vi "RobotDriveOpen6MotorWithTalonSRX.vi"(0 "Left Motor 1":u8=255, 1 "Left Motor 2":u8=255, 2 "Left Motor 3":u8=255, 3 "Right Motor 1":u8=255, 4 "Right Motor 2":u8=255, 5 "Right Motor 3":u8=255, 7 "error in (no error)":errorcluster, 8 "Left Motor 1 Inverted":bool, 9 "Right Motor 1 Inverted":bool, 10 "Left Motor 2 Inverted":bool, 11 "Right Motor 2 Inverted":bool, 12 "Left Motor 3 Inverted":bool, 13 "Right Motor 3 Inverted":bool) -> (20 "RobotDriveDevRef":T1={"DevStatus"={"status"=FALSE, "code"=0, "source"=""}, "Motors[]"=[], "Square Inputs"=FALSE, "Max Output"=1.0}, 27 "error out":errorcluster)   [LabVIEW 2017, in "ArgosLib.lvlib"]
doc: "Opens a reference to the robot drive for a two-, four-, or six-motor robot using Talon SR motor controllers connected via CAN bus.\n\nFor 2-motor drive, connect Left Motor 1 and Right Motor 1.\nFor 4-motor drive, connect Left Motor 2 and Right Motor 2 in addition to the 2-motor drive connections.\nFor 6-motor drive, connect Left Motor 3 and Right Motor 3 in addition to the 4-motor drive connections.\n\nInversions are optional and are set to false if disconnected.\n\nThis software is licensed. Open the labview\\readme\\WPI Robotics Library Open Source License.txt file for more information."
uses:
  ArgosLib.lvlib
  <vilib>/Rock Robotics/WPI/RobotDrive/WPI_RobotDriveDevRef.ctl
  <vilib>/Rock Robotics/WPI/MotorControl/WPI_MotorControlDeviceRef.ctl
  <vilib>/Rock Robotics/WPI/MotorControl/WPI_MotorControlType.ctl
  <vilib>/Rock Robotics/SystemInterfaces/DIO/FPGA_DIOPWMChannel.ctl
  <vilib>/Rock Robotics/WPI/PWM/WPI_PWMDeadband.ctl
  <vilib>/Rock Robotics/SystemInterfaces/DIO/FPGA_DIOChannel.ctl
  <vilib>/Rock Robotics/WPI/SafetyOutput/WPI_SafetyOutputConfigMenu.ctl
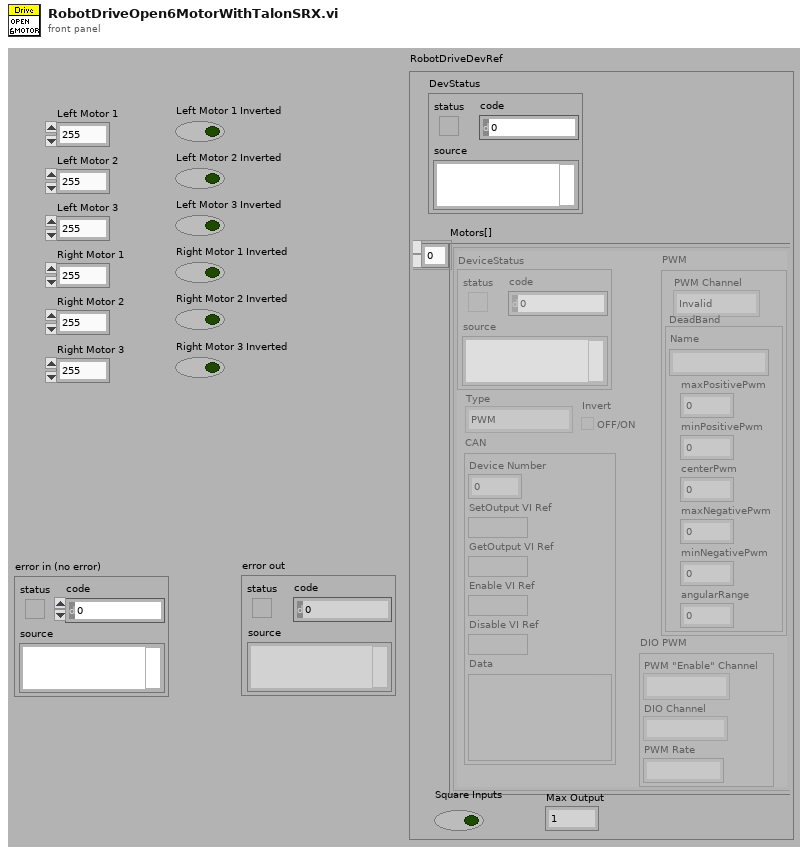
[diagram p1: front panel]
types:
  T1 = typedef "WPI_RobotDriveDevRef.ctl" = cluster{"DevStatus":errorcluster, "Motors[]":T2[], "Square Inputs":bool, "Max Output":dbl}
  T2 = typedef "WPI_MotorControlDeviceRef.ctl" = cluster{"DeviceStatus":errorcluster, "Type":T3, "PWM":cluster{"PWM Channel":T4, "DeadBand":T5}, "CAN":cluster{"Device Number":u8, "SetOutput VI Ref":variant, "GetOutput VI Ref":variant, "Enable VI Ref":variant, "Disable VI Ref":variant, "Data":variant}, "Invert":bool, "DIO PWM":cluster{"PWM \"Enable\" Channel":T4, "DIOChannel":T6, "PWM Rate":dbl}}
  T3 = typedef "WPI_MotorControlType.ctl" = enum16{"PWM", "CAN", "DIO PWM"}
  T4 = typedef "FPGA_DIOPWMChannel.ctl" = enum8{"PWM 0", "PWM 1", "PWM 2", "PWM 3", "PWM 4", "PWM 5", "PWM 6", "PWM 7", "PWM 8", "PWM 9", "PWM MXP 0", "PWM MXP 1", "PWM MXP 2", "PWM MXP 3", "PWM MXP 4", "PWM MXP 5", "PWM MXP 6", "PWM MXP 7", "PWM MXP 8", "PWM MXP 9", "Invalid"}
  T5 = typedef "WPI_PWMDeadband.ctl" = cluster{"Name":string, "maxPositivePwm":i32, "minPositivePwm":i32, "centerPwm":i32, "maxNegativePwm":i32, "minNegativePwm":i32, "angularRange":u16}
  T6 = typedef "FPGA_DIOChannel.ctl" = enum8{"DIO 0", "DIO 1", "DIO 2", "DIO 3", "DIO 4", "DIO 5", "DIO 6", "DIO 7", "DIO 8", "DIO 9", "DIO MXP 0", "DIO MXP 1", "DIO MXP 2", "DIO MXP 3", "DIO MXP 4", "DIO MXP 5", "DIO MXP 6", "DIO MXP 7", "DIO MXP 8", "DIO MXP 9", "DIO MXP 10", "DIO MXP 11", "DIO MXP 12", "DIO MXP 13", "DIO MXP 14", "DIO MXP 15", "SPI Port CS1", "SPI Port CS2", "SPI Port CS3", "SPI Port MISO", "SPI Port MOSI", "Invalid"}
  T7 = typedef "WPI_SafetyOutputConfigMenu.ctl" = enum16{"Enable", "Disable"}
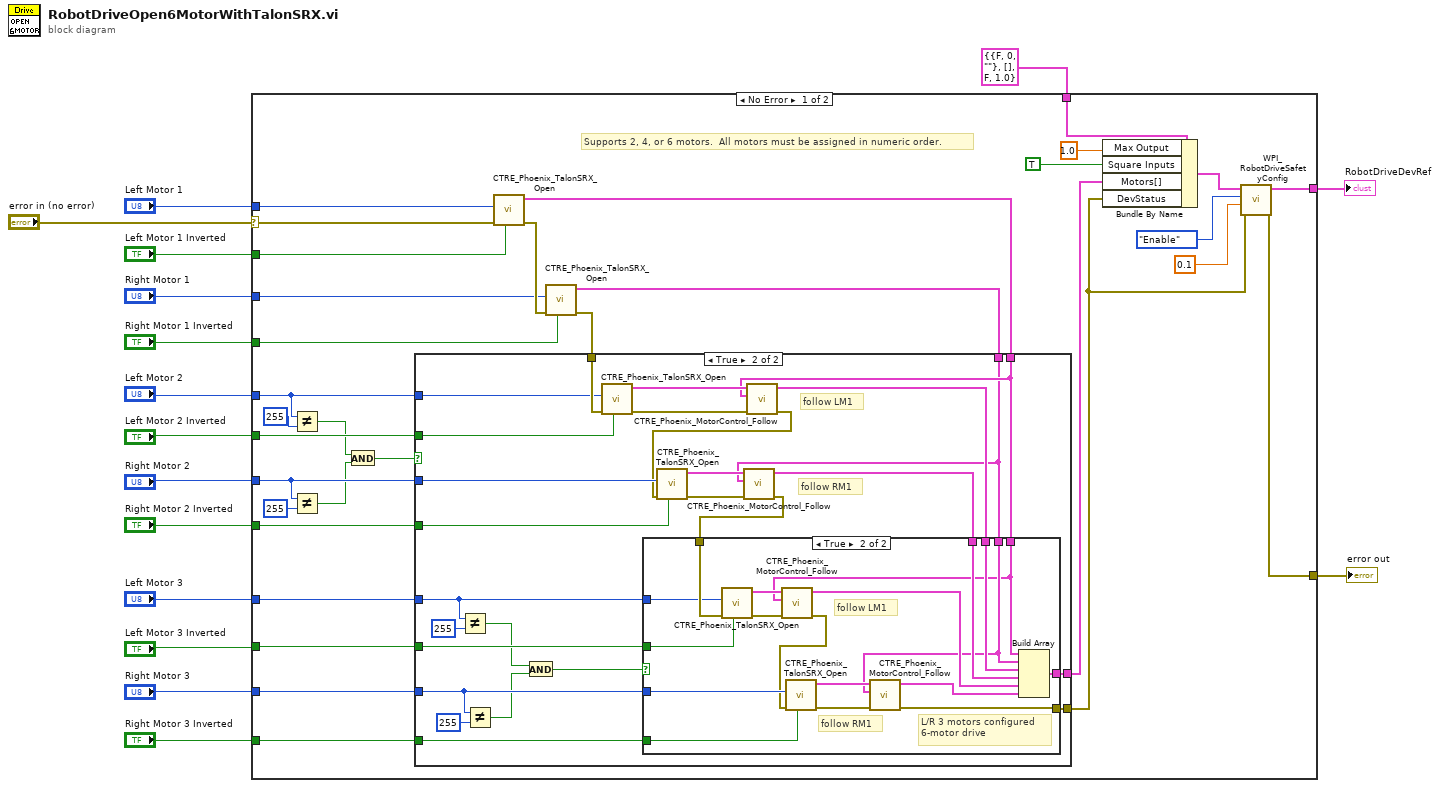
[diagram p0: block diagram]
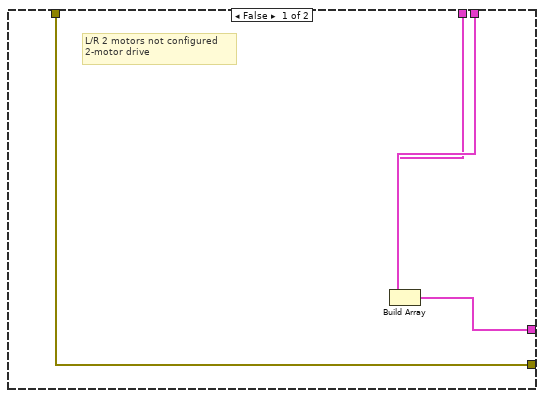
[diagram p2: hidden frame]
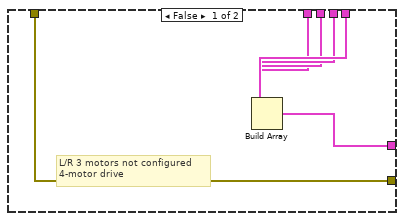
[diagram p3: hidden frame]
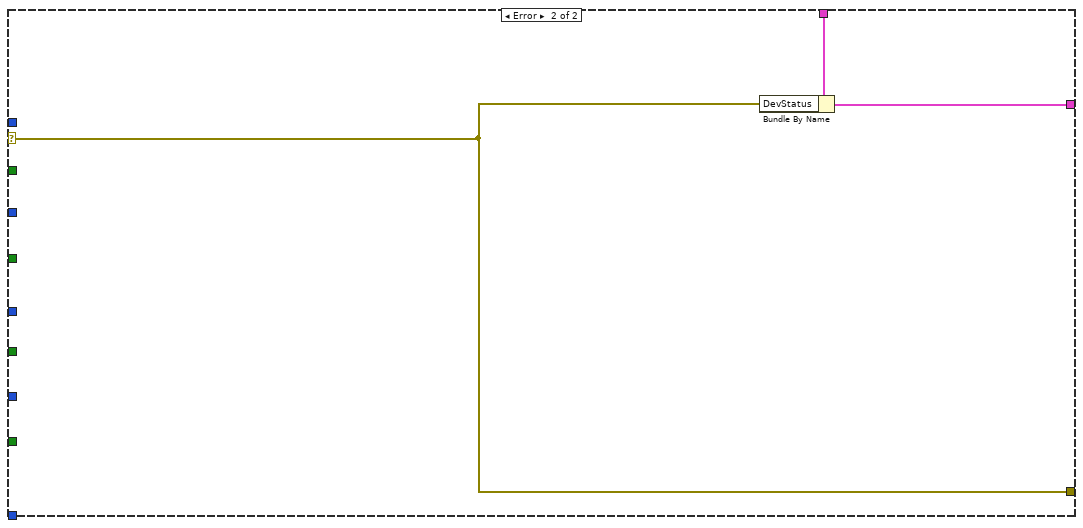
[diagram p4: hidden frame]
diagram:
  n1 = case shown="No Error" "error in (no error)" {
    selector: "error in (no error)" -> [w27 w103]
    tunnel: [w37 w104] -> w16
    tunnel: T1 {"DevStatus"={"status"=FALSE, "code"=0, "source"=""}, "Motors[]"=[], "Square Inputs"=FALSE, "Max Output"=1.0} ("RobotDriveDevRef") -> [w48 w105]
    tunnel: "Left Motor 1 Inverted" -> [w44 _]
    tunnel: "Right Motor 1 Inverted" -> [w43 _]
    tunnel: "Right Motor 2 Inverted" -> [w41 _]
    tunnel: "Left Motor 2 Inverted" -> [w42 _]
    tunnel: [w38 w103] -> w9
    tunnel: "Left Motor 3 Inverted" -> [w34 _]
    tunnel: "Right Motor 3 Inverted" -> [w33 _]
    tunnel: "Left Motor 1" -> [w31 _]
    tunnel: "Right Motor 1" -> [w30 _]
    tunnel: "Left Motor 2" -> [w26 _]
    tunnel: "Right Motor 2" -> [w23 _]
    tunnel: "Left Motor 3" -> [w29 _]
    tunnel: "Right Motor 3" -> [w28 _]
    frame No Error {
      # "Supports 2, 4, or 6 motors.  All motors must be assigned in numeric order."
      n2 = Not Equal?(x=w26, y=u8 255) -> (x != y?=w22:bool)
      n3 = Not Equal?(x=w23, y=u8 255) -> (x != y?=w21:bool)
      n4 = And(x=w22, y=w21) -> (x .and. y?=w20:bool)
      n5 = call <vilib>:"CTRE_Phoenix_TalonSRX_Open.vi"("Invert"=w44, "error in"=w27, "Device Number"=w31) -> ("error out"=w45:errorcluster, "CAN Talon SRX Ref"=w17:T2)  [unwired: 7 in]
      n6 = call <vilib>:"CTRE_Phoenix_TalonSRX_Open.vi"("Invert"=w43, "error in"=w45, "Device Number"=w30) -> ("error out"=w46:errorcluster, "CAN Talon SRX Ref"=w18:T2)  [unwired: 7 in]
      n7 = case shown="True" w20 {
        tunnel: w46 -> [w52 w78]
        tunnel: w42 -> [_ w77]
        tunnel: w41 -> [_ w76]
        tunnel: w34 -> [_ w75]
        tunnel: w33 -> [_ w74]
        tunnel: [w52 w73] -> w32
        tunnel: w29 -> [_ w67]
        tunnel: w28 -> [_ w68]
        tunnel: w26 -> [_ w72]
        tunnel: w23 -> [_ w71]
        tunnel: [w51 w63] -> w19
        tunnel: w17 -> [w50 w58]
        tunnel: w18 -> [w49 w53]
        frame False {
          # "L/R 2 motors not configured\n2-motor drive"
          n8 = Build Array(w50, w49) -> (w51:T2[])
        }
        frame True {
          # "follow LM1"
          # "follow RM1"
          n9 = Not Equal?(x=w67, y=u8 255) -> (x != y?=w65:bool)
          n10 = Not Equal?(x=w68, y=u8 255) -> (x != y?=w64:bool)
          n11 = And(x=w65, y=w64) -> (x .and. y?=w66:bool)
          n12 = call <vilib>:"CTRE_Phoenix_TalonSRX_Open.vi"("Invert"=w77, "error in"=w78, "Device Number"=w72) -> ("error out"=w60:errorcluster, "CAN Talon SRX Ref"=w62:T2)  [unwired: 7 in]
          n13 = call <vilib>:"CTRE_Phoenix_MotorControl_Follow.vi"("error in (no error)"=w60, "Master Controller to Follow"=w58, "PhoenixMotorControlDevRef"=w62) -> ("error out"=w59:errorcluster, "PhoenixMotorControlDevRef"=w61:T2)  [unwired: 7 in]
          n14 = call <vilib>:"CTRE_Phoenix_TalonSRX_Open.vi"("Invert"=w76, "error in"=w59, "Device Number"=w71) -> ("error out"=w55:errorcluster, "CAN Talon SRX Ref"=w57:T2)  [unwired: 7 in]
          n15 = call <vilib>:"CTRE_Phoenix_MotorControl_Follow.vi"("error in (no error)"=w55, "Master Controller to Follow"=w53, "PhoenixMotorControlDevRef"=w57) -> ("error out"=w54:errorcluster, "PhoenixMotorControlDevRef"=w56:T2)  [unwired: 7 in]
          n16 = case shown="True" w66 {
            tunnel: w54 -> [w84 w102]
            tunnel: w75 -> [_ w101]
            tunnel: w74 -> [_ w100]
            tunnel: [w84 w86] -> w73
            tunnel: w67 -> [_ w99]
            tunnel: w68 -> [_ w98]
            tunnel: [w83 w97] -> w63
            tunnel: w58 -> [w82 w85]
            tunnel: w53 -> [w81 w88]
            tunnel: w61 -> [w80 w96]
            tunnel: w56 -> [w79 w95]
            frame False {
              # "L/R 3 motors not configured\n4-motor drive"
              n17 = Build Array(w82, w81, w80, w79) -> (w83:T2[])
            }
            frame True {
              # "follow LM1"
              # "follow RM1"
              # "L/R 3 motors configured\n6-motor drive"
              n18 = call <vilib>:"CTRE_Phoenix_TalonSRX_Open.vi"("Invert"=w101, "error in"=w102, "Device Number"=w99) -> ("error out"=w92:errorcluster, "CAN Talon SRX Ref"=w94:T2)  [unwired: 7 in]
              n19 = call <vilib>:"CTRE_Phoenix_MotorControl_Follow.vi"("error in (no error)"=w92, "Master Controller to Follow"=w85, "PhoenixMotorControlDevRef"=w94) -> ("error out"=w91:errorcluster, "PhoenixMotorControlDevRef"=w93:T2)  [unwired: 7 in]
              n20 = call <vilib>:"CTRE_Phoenix_TalonSRX_Open.vi"("Invert"=w100, "error in"=w91, "Device Number"=w98) -> ("error out"=w87:errorcluster, "CAN Talon SRX Ref"=w90:T2)  [unwired: 7 in]
              n21 = call <vilib>:"CTRE_Phoenix_MotorControl_Follow.vi"("error in (no error)"=w87, "Master Controller to Follow"=w88, "PhoenixMotorControlDevRef"=w90) -> ("error out"=w86:errorcluster, "PhoenixMotorControlDevRef"=w89:T2)  [unwired: 7 in]
              n22 = Build Array(w85, w88, w96, w95, w93, w89) -> (w97:T2[])
            }
          }
        }
      }
      n23 = Bundle By Name(cluster=w48, "Max Output"=1.0, "Square Inputs"=TRUE ("DestroyPWM?"), "Motors[]"=w19, "DevStatus"=w32) -> (w39:T1)
      n24 = call <vilib>:"WPI_RobotDriveSafetyConfig.vi"("error in (no error)"=w32, "timeout (s)"=0.1, "mode"=WPI_SafetyOutputConfigMenu."Enable", "RobotDriveDevRef"=w39) -> ("error out"=w38:errorcluster, "RobotDriveDevRef"=w37:T1)  [unwired: 6 out]
    }
    frame Error {
      n25 = Bundle By Name(cluster=w105, "DevStatus"=w103) -> (w104:T1)
    }
  }
  "RobotDriveDevRef" <- w16
  "error out" <- w9
